vi "Programa_robot_final_6.vi"() -> ()   [LabVIEW 2019]
uses:
  <vilib>/Instr/_visa.llb/VISA Configure Serial Port (Instr).vi
  Global_STOP.vi
  <vilib>/regexp/Match Regular Expression.xnode
panel:
  in  "stop socket 3":bool
  in  "Ruta hacia el fichero que contiene la imagen de la       superficie del ASIC  fotografiada por la camara en el bloque de borrado de la imagen previa capturada":path=path "C:/Trabajo_Robot/Test Asic Javi_2021/Origen Socket SERVO_PCB_BUENO_v5 (muchos asics)/capturaQR.jpg"
  in  "stop 6":bool
  in  "Abrir socket 2":bool
  in  "Cerrar socket 2":bool
  in  "Interruptor Error 2":bool
  in  "stop 5":bool
  out "Datos_QR 3":string
  out "Existe foto anterior?":bool
  in  "STOP TEST 3":bool
  in  "Interruptor Error":bool
  in  "Cerrar socket":bool
  in  "Abrir socket":bool
  out "Error_QR":bool
  out "return count":u32
  out "lectura puerto serie":u32
  out "dato escrito puerto serie":string
  out "TEST OK":bool
  out "error out":errorcluster {"code" format="%f"}
  in  "STOP TEST 2":bool
  out "Datos_QR 2":string
  out "NUMERO ASICS TESTEADOS":i32
  in  "Config File":path=path "C:/Trabajo_Robot/Test Asic Javi_2021/Origen Socket SERVO_PCB_BUENO_v5 (muchos asics)/CONFIG/configuracion_robot_CTAV2022A.test"
  in  "SELECCION DE TEST":string(combo)="COMPLETO"
  in  "?":bool
  out "Boolean":bool
  in  "stop socket 2":bool
  out "Bytes at port 3":u32=1
  in  "IN y":string(combo)="00"
  in  "IN x":string(combo)="00"
  in  "NOK y":string(combo)="00"
  in  "NOK x":string(combo)="00"
  in  "OK y":string(combo)="00"
  in  "OK x":string(combo)="00"
  in  "Operator's name":string(combo)="Juan Rodríguez"
  in  "?":bool
  in  "Fichero de registro":path=path "C:/Trabajo_Robot/Pruebas/Pruebas.txt"
  in  "Path Out Report":path=path "C:/Trabajo_Robot/desde Marzo 2023/Pruebas_PC_APD/RESULT_TEST_C_LABP0/Test_33_ASIC_Referencia"
  in  "stop socket":bool
  out "Bytes at port 1":u32
  out "Iteraciones":i32
  out "Lectura buffer":string="1"
  in  "Delay (ms)":dbl=1.0 min=1.0 max=9.0 step=1.0
  out "Bytes at port 2":u32=1
  in  "Interruptor":bool=TRUE
  in  "stop":bool
  # "SI SE PRESIONA EL BOTON STOP PARA INTERRUMPIR EL TEST,\nHAY QUE APAGAR Y VOLVER A ENCENDER EL ARDUINO\nCON EL SWITCH DE LA CAJA."
  # "x: columna en cada bandeja \ny: fila en cada bandeja"
  # "Funcionamiento: en la primera iteración, el efector se desplaza desde el origen hasta la celda\nintroducida, hace una pausa, va a la posición del socket (0,0), hace otra pausa, va a la celda\nde salida y vuelve al origen. En las iteraciones siguientes hará lo mismo pero recorriendo las\nceldas de la bandeja sucesivamente. Que el desplazamiento se produzca hacia una celda de\nla bandeja OK o de la bandeja NOK depende de la salidad del programa de test de Asics."
types:
  T1 = enum16{"open", "replace", "create", "open or create", "replace or create", "replace or create with confirmation"}
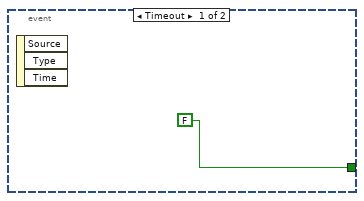
[diagram p2: hidden frame]
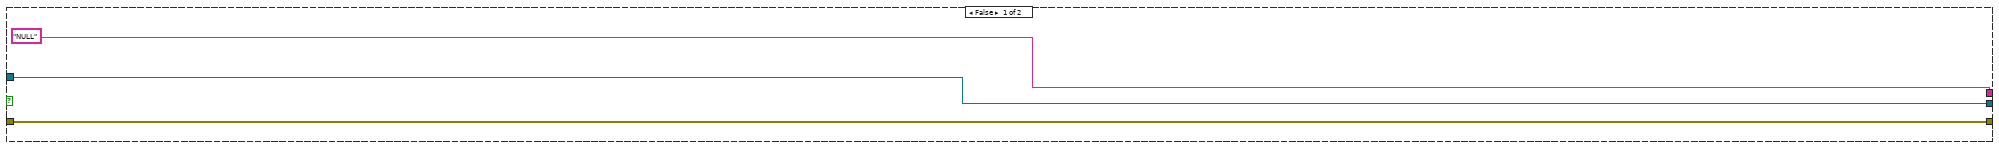
[diagram p5: hidden frame]
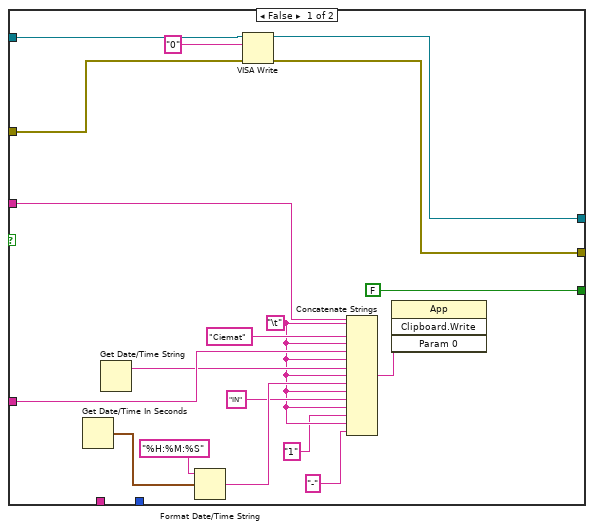
[diagram p9: hidden frame]
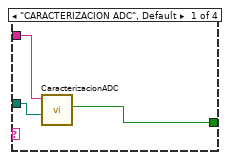
[diagram p10: hidden frame]
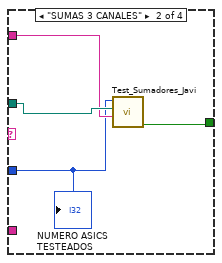
[diagram p11: hidden frame]
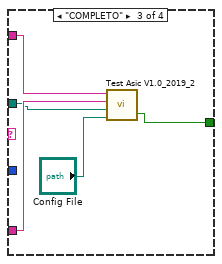
[diagram p12: hidden frame]
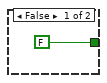
[diagram p13: hidden frame]
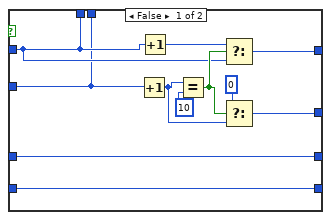
[diagram p15: hidden frame]
diagram:
  n1 = control-ref of="stop socket"() -> (w1:refnum<vi>)
  n2 = control-ref of="Cerrar socket"() -> (w9:refnum<vi>)
  n3 = control-ref of="STOP TEST 2"() -> (w12:refnum<vi>)
  n4 = control-ref of="Abrir socket"() -> (w7:refnum<vi>)
  n5 = control-ref of="stop"() -> (w8:refnum<vi>)
  n6 = control-ref of="Interruptor Error"() -> (w10:refnum<vi>)
  n7 = property class="Bool (strict)"(reference=w12, "Visible"=FALSE) -> ()  [unwired: 1 in, 2 out]
  n8 = property class="Bool (strict)"(reference=w7, "Visible"=FALSE) -> ()  [unwired: 1 in, 2 out]
  n9 = property class="Bool (strict)"(reference=w10, "Visible"=FALSE) -> ()  [unwired: 1 in, 2 out]
  n10 = property class="Bool (strict)"(reference=w9, "Visible"=FALSE) -> ()  [unwired: 1 in, 2 out]
  n11 = property on="Boolean" class="Bool (strict)"("Visible"=FALSE) -> ()  [unwired: 2 in, 2 out]
  n12 = property class="Bool"(reference=w1, "Visible"=FALSE) -> ()  [unwired: 1 in, 2 out]
  n13 = property class="Bool"(reference=w8, "Visible"=FALSE) -> ()  [unwired: 1 in, 2 out]
  n14 = flat-sequence {
    tunnel: [w54] -> w18
    tunnel: ["Fichero de registro"] -> w17
    tunnel: ["SELECCION DE TEST"] -> w16
    tunnel: ["NOK y"] -> w33
    tunnel: ["NOK x"] -> w32
    tunnel: ["OK y"] -> w31
    tunnel: ["OK x"] -> w30
    tunnel: ["IN y"] -> w29
    tunnel: ["IN x"] -> w28
    tunnel: [w57] -> w27
    tunnel: [w58] -> w26
    tunnel: ["IN y"] -> w25
    tunnel: ["IN x"] -> w24
    tunnel: w17 -> [w56]
    frame #0 {
      n15 = while {
        stop <- "?" stop-if-true
        n16 = Not(x="?") -> (.not. x?=w50:bool)
        "Boolean" <- w50
        n17 = property on="Boolean" class="Bool (strict)"("Blinking"=w50) -> ()  [unwired: 2 in, 2 out]
      }
      n18 = global write "Global_STOP.vi" "stop"(FALSE ("stop")) -> ()
    }
    frame #1 {
      n19 = Not(x="?") -> (.not. x?=w54:bool)
    }
    frame #2 {
      n20 = Open/Create/Replace File(file path (use dialog)=w56, operation (0:open)=T1."open", access (0:read/write)=enum16{"read/write", "read-only", "write-only"}."write-only") -> (refnum out=w69:refnum<file>, error out=w71:errorcluster)  [unwired: 3 in, 1 out]
      n21 = Set File Position(refnum=w69, from (0:start)=enum16{"start", "end", "current"}."end", error in=w71) -> (refnum out=w70:refnum<file>, error out=w72:errorcluster)  [unwired: 1 in]
      n22 = Write to Text File(file (use dialog)=w70, text="\r\n", error in=w72) -> (refnum out=w58:refnum<file>, error out=w57:errorcluster)  [unwired: 1 in, 1 out]
    }
  }
  n23 = Decimal String To Number(string=w25) -> (number=w23:i32)  [unwired: 2 in, 1 out]
  n24 = Decimal String To Number(string=w24) -> (number=w20:i32)  [unwired: 2 in, 1 out]
  n25 = Multiply(x=10, y=w23) -> (x*y=w21:i32)
  n26 = Decimal String To Number(string=w31) -> (number=w35:i32)  [unwired: 2 in, 1 out]
  n27 = Decimal String To Number(string=w30) -> (number=w34:i32)  [unwired: 2 in, 1 out]
  n28 = Decimal String To Number(string=w33) -> (number=w37:i32)  [unwired: 2 in, 1 out]
  n29 = Decimal String To Number(string=w32) -> (number=w36:i32)  [unwired: 2 in, 1 out]
  n30 = call-poly "VISA Configure Serial Port"("VISA resource name"=refnum<visa-resource-name> "COM9", "baud rate (9600)"=u32 9600, "data bits (8)"=u16 8) -> ("VISA resource name out"=w41:refnum<visa-resource-name>, "error out"=w44:errorcluster)  [unwired: 11 in]
  n31 = Add(x=w21, y=w20) -> (x+y=w19:i32)
  n32 = while {
    shift-right: [w87] -> w42
    shift-left: w44 -> [w126]
    tunnel: w41 -> [w124]
    tunnel: [w89] -> w43
    tunnel: w26 -> [w117]
    tunnel: [w116] -> w40
    tunnel: w27 -> [w115]
    tunnel: [w114] -> w39
    tunnel: w28 -> [w112]
    tunnel: w29 -> [w111]
    tunnel: w30 -> [w110]
    tunnel: w31 -> [w109]
    tunnel: w32 -> [w108]
    tunnel: w33 -> [w107]
    shift-right: [w100] -> _
    shift-left: w37 -> [w106]
    shift-right: [w102] -> _
    shift-left: w36 -> [w105]
    shift-right: [w99] -> _
    shift-left: w35 -> [w104]
    shift-right: [w101] -> _
    shift-left: w34 -> [w103]
    tunnel: w19 -> [w77]
    tunnel: w18 -> [w91]
    tunnel: w16 -> [w90]
    tunnel: [w78] -> w14
    i -> [w73]
    stop <- w74 stop-if-true
    # "Cuando Arduino deja un ASIC en la bandeja de  entrada ó en las de OK/NOK\ny vuelve a la posicion de socket, envia un \"2\" por el puerto serie\na labview y éste lo lee para que se salga del bucle, y prosiga la secuencia que le queda\nal programa, para después coger otro asic. Javier Morales"
    n33 = flat-sequence {
      tunnel: w126 -> [w179]
      tunnel: w124 -> [w168]
      tunnel: [w170] -> w123
      tunnel: [w169] -> w122
      tunnel: w112 -> [w149]
      tunnel: w111 -> [w148]
      tunnel: w110 -> [w147]
      tunnel: w109 -> [w146]
      tunnel: w108 -> [w145]
      tunnel: w107 -> [w144]
      tunnel: w123 -> [w916]
      tunnel: w122 -> [w915]
      tunnel: [w914] -> w98
      tunnel: [w913] -> w96
      tunnel: [w912] -> _
      tunnel: w98 -> [w933]
      tunnel: [w931] -> w97
      tunnel: w96 -> [w932]
      tunnel: [w930] -> w95
      tunnel: w97 -> [w954]
      tunnel: w95 -> [w953]
      tunnel: w73 -> [w955]
      tunnel: [w951] -> w94
      tunnel: [w950] -> w93
      tunnel: [w949] -> w92
      tunnel: w73 -> [w1071]
      tunnel: [w1073] -> w120
      tunnel: [w1072] -> w119
      tunnel: [w1069] -> w113
      tunnel: w94 -> [w1068]
      tunnel: w93 -> [w1067]
      tunnel: w92 -> [w1066]
      tunnel: w91 -> [w1061]
      tunnel: w90 -> [w1064]
      tunnel: w73 -> [w1063]
      tunnel: [w1141] -> w118
      tunnel: [w1143] -> w121
      tunnel: w120 -> [w1142]
      tunnel: w119 -> [w1140]
      tunnel: w117 -> [w1147]
      tunnel: [w1146] -> w116
      tunnel: w115 -> [w1145]
      tunnel: [w1144] -> w114
      tunnel: w73 -> [w1137]
      tunnel: w113 -> [w1136]
      tunnel: w106 -> [w1132]
      tunnel: w105 -> [w1135]
      tunnel: w104 -> [w1134]
      tunnel: w103 -> [w1133]
      tunnel: [w1131] -> w100
      tunnel: [w1130] -> w102
      tunnel: [w1129] -> w99
      tunnel: [w1128] -> w101
      tunnel: w77 -> [w1127]
      tunnel: w73 -> [w1126]
      tunnel: [w1125] -> _
      frame #0 {
        n34 = for {
          N: 2 -> [_]
          shift-right: [w791] -> _
          shift-left: w149 -> [w796]
          shift-right: [w794] -> w165
          shift-left: w168 -> [w795]
          shift-right: [w792] -> w164
          shift-left: w179 -> [w793]
          n35 = xnode "Match Regular Expression"("input string"=w796, "regular expression"="-?\\d") -> ("whole match"=w790:string, "after match"=w791:string)  [unwired: 4 in, 3 out]
          n36 = VISA Write(VISA resource name=w795, write buffer=w790, error in (no error)=w793) -> (VISA resource name out=w794:refnum<visa-resource-name>, error out=w792:errorcluster)  [unwired: 1 out]
        }
        n37 = for {
          N: 2 -> [_]
          shift-right: [w669] -> _
          shift-left: w148 -> [w674]
          shift-right: [w672] -> w159
          shift-left: w165 -> [w673]
          shift-right: [w670] -> w158
          shift-left: w164 -> [w671]
          n38 = xnode "Match Regular Expression"("input string"=w674, "regular expression"="-?\\d") -> ("whole match"=w668:string, "after match"=w669:string)  [unwired: 4 in, 3 out]
          n39 = VISA Write(VISA resource name=w673, write buffer=w668, error in (no error)=w671) -> (VISA resource name out=w672:refnum<visa-resource-name>, error out=w670:errorcluster)  [unwired: 1 out]
        }
        n40 = for {
          N: 2 -> [_]
          shift-right: [w547] -> _
          shift-left: w147 -> [w552]
          shift-right: [w550] -> w161
          shift-left: w159 -> [w551]
          shift-right: [w548] -> w160
          shift-left: w158 -> [w549]
          n41 = xnode "Match Regular Expression"("input string"=w552, "regular expression"="-?\\d") -> ("whole match"=w546:string, "after match"=w547:string)  [unwired: 4 in, 3 out]
          n42 = VISA Write(VISA resource name=w551, write buffer=w546, error in (no error)=w549) -> (VISA resource name out=w550:refnum<visa-resource-name>, error out=w548:errorcluster)  [unwired: 1 out]
        }
        n43 = for {
          N: 2 -> [_]
          shift-right: [w425] -> _
          shift-left: w146 -> [w430]
          shift-right: [w428] -> w153
          shift-left: w161 -> [w429]
          shift-right: [w426] -> w152
          shift-left: w160 -> [w427]
          n44 = xnode "Match Regular Expression"("input string"=w430, "regular expression"="-?\\d") -> ("whole match"=w424:string, "after match"=w425:string)  [unwired: 4 in, 3 out]
          n45 = VISA Write(VISA resource name=w429, write buffer=w424, error in (no error)=w427) -> (VISA resource name out=w428:refnum<visa-resource-name>, error out=w426:errorcluster)  [unwired: 1 out]
        }
        n46 = for {
          N: 2 -> [_]
          shift-right: [w303] -> _
          shift-left: w145 -> [w308]
          shift-right: [w306] -> w155
          shift-left: w153 -> [w307]
          shift-right: [w304] -> w154
          shift-left: w152 -> [w305]
          n47 = xnode "Match Regular Expression"("input string"=w308, "regular expression"="-?\\d") -> ("whole match"=w302:string, "after match"=w303:string)  [unwired: 4 in, 3 out]
          n48 = VISA Write(VISA resource name=w307, write buffer=w302, error in (no error)=w305) -> (VISA resource name out=w306:refnum<visa-resource-name>, error out=w304:errorcluster)  [unwired: 1 out]
        }
        n49 = for {
          N: 2 -> [_]
          shift-right: [w181] -> _
          shift-left: w144 -> [w186]
          shift-right: [w184] -> w151
          shift-left: w155 -> [w185]
          shift-right: [w182] -> w150
          shift-left: w154 -> [w183]
          n50 = xnode "Match Regular Expression"("input string"=w186, "regular expression"="-?\\d") -> ("whole match"=w180:string, "after match"=w181:string)  [unwired: 4 in, 3 out]
          n51 = VISA Write(VISA resource name=w185, write buffer=w180, error in (no error)=w183) -> (VISA resource name out=w184:refnum<visa-resource-name>, error out=w182:errorcluster)  [unwired: 1 out]
        }
        n52 = Number To Decimal String(number="Delay (ms)") -> (decimal integer string=w173:string)  [unwired: 1 in]
        n53 = VISA Write(VISA resource name=w151, write buffer=w173, error in (no error)=w150) -> (VISA resource name out=w175:refnum<visa-resource-name>, error out=w174:errorcluster)  [unwired: 1 out]
        n54 = Select(t="1" ("write buffer"), s="Interruptor", f="0" ("write buffer")) -> (s? t:f=w171:string)
        n55 = VISA Write(VISA resource name=w175, write buffer=w171, error in (no error)=w174) -> (VISA resource name out=w170:refnum<visa-resource-name>, error out=w169:errorcluster)  [unwired: 1 out]
      }
      frame #1 {
        n56 = while {
          shift-right: [w923] -> w913
          shift-left: w915 -> [w928]
          tunnel: ["stop socket"] -> _
          shift-right: [w924] -> w914
          shift-left: w916 -> [w929]
          tunnel: ["stop socket"] -> w912
          stop <- w918 stop-if-true
          n57 = property class="Instr"(reference=w929, error in=w928) -> (reference out=w927:refnum<visa-resource-name>, error out=w926:errorcluster, "Bytes at Port"=w925:u32)
          "Bytes at port 1" <- w925
          n58 = VISA Read(VISA resource name=w927, byte count=w925, error in (no error)=w926) -> (VISA resource name out=w924:refnum<visa-resource-name>, read buffer=w922:string, error out=w923:errorcluster)  [unwired: 1 out]
          n59 = Equal?(x="2", y=w922) -> (x = y?=w920:bool)
          n60 = global read "Global_STOP.vi" "stop"() -> (w917:bool)
          n61 = Compound Arithmetic op=OR(w920, "stop socket", w917) -> (w918:bool)
        }
      }
      frame #2 {
        n62 = while {
          shift-right: [w940] -> w930
          shift-left: w932 -> [w945]
          tunnel: ["stop socket 2"] -> _
          shift-right: [w941] -> w931
          shift-left: w933 -> [w946]
          tunnel: ["stop socket 2"] -> _
          stop <- w935 stop-if-true
          n63 = property class="Instr"(reference=w946, error in=w945) -> (reference out=w944:refnum<visa-resource-name>, error out=w943:errorcluster, "Bytes at Port"=w942:u32)
          "Bytes at port 3" <- w942
          n64 = VISA Read(VISA resource name=w944, byte count=w942, error in (no error)=w943) -> (VISA resource name out=w941:refnum<visa-resource-name>, read buffer=w939:string, error out=w940:errorcluster)  [unwired: 1 out]
          n65 = Equal?(x="3", y=w939) -> (x = y?=w937:bool)
          n66 = global read "Global_STOP.vi" "stop"() -> (w934:bool)
          n67 = Compound Arithmetic op=OR(w937, "stop socket 2", w934) -> (w935:bool)
        }
      }
      frame #3 {
        # "Este bloque realiza la captura y lectura del QR"
        n68 = Greater?(x=w955, y=-1) -> (0:w952:bool)
        n69 = case shown="True" w952 {
          tunnel: [w959 w962] -> w949
          tunnel: w954 -> [w959 w964]
          tunnel: [w958 w963] -> w951
          tunnel: w953 -> [w958 w965]
          tunnel: ["NULL" ("Datos_QR") w961] -> w950
          frame False {
          }
          frame True {
            n70 = property on="Error_QR" class="Bool (strict)"("Value"=FALSE ("Error_QR")) -> ()  [unwired: 2 in, 2 out]
            n71 = while {
              tunnel: [w972] -> w961
              tunnel: w964 -> [w982]
              tunnel: [w978] -> w962
              tunnel: [w977] -> w963
              tunnel: w965 -> [w973]
              stop <- w970 stop-if-true
              n72 = flat-sequence {
                tunnel: [w986] -> w974
                tunnel: w973 -> [w984]
                tunnel: [w998] -> w972
                tunnel: [w997] -> w967
                tunnel: w974 -> [w996]
                tunnel: [w996] -> w968
                frame #0 {
                  # "Éste bloque borra el fichero de imagen\ndel Asic anterior."
                  n73 = call <vilib>:"Check if File or Folder Exists.vi"("error in (no error)"=w984, "path"="Ruta hacia el fichero que contiene la imagen de la       superficie del ASIC  fotografiada por la camara en el bloque de borrado de la imagen previa capturada") -> ("error out"=w985:errorcluster, "file or folder exists?"=w988:bool, "dup path"=w987:path)  [unwired: 7 in]
                  "Existe foto anterior?" <- w988
                  n74 = case shown="True" w988 {
                    tunnel: w987 -> [w990 w994]
                    tunnel: [w990 w993] -> _
                    tunnel: [w989 w992] -> w986
                    tunnel: w985 -> [w989 w991]
                    frame False {
                    }
                    frame True {
                      n75 = Delete(path (use dialog)=w994, error in=w991) -> (deleted path=w993:path, error out=w992:errorcluster)  [unwired: 3 in, 1 out]
                    }
                  }
                }
                frame #1 {
                  # "Éste bloque realiza la captura de imagen\ndel QR del Asic para leer el código."
                  n76 = for {
                    N: 5 -> [_]
                    tunnel: [w1003] -> w998
                    tunnel: [w1001] -> w997
                    stop <- w999 stop-if-true
                    n77 = call "CapturaImagenyQR_subVI_pruebas.vi"() -> ("Datos_QR"=w1003:string)  [unwired: 11 in]
                    "Datos_QR 3" <- w1003
                    n78 = Equal?(x=w1003, y="" ("Datos_QR")) -> (x = y?=w1002:bool)
                    n79 = global read "Global_STOP.vi" "stop"() -> (w1000:bool)
                    n80 = Not(x=w1002) -> (.not. x?=w1001:bool)
                    n81 = Compound Arithmetic op=OR(w1001, w1000) -> (w999:bool)
                  }
                }
              }
              n82 = Not(x=w967) -> (.not. x?=w969:bool)
              "Error_QR" <- w969
              n83 = Select(t="1" ("write buffer"), s=w967, f="0" ("write buffer")) -> (s? t:f=w979:string)
              n84 = VISA Write(VISA resource name=w982, write buffer=w979, error in (no error)=w968) -> (VISA resource name out=w976:refnum<visa-resource-name>, error out=w975:errorcluster)  [unwired: 1 out]
              n85 = global read "Global_STOP.vi" "stop"() -> (w971:bool)
              n86 = case shown="False" w967 {
                tunnel: w976 -> [w1016 w1057]
                tunnel: w975 -> [w1015 w1056]
                tunnel: [w1014 w1057] -> w978
                tunnel: [w1013 w1056] -> w977
                frame False {
                  n87 = flat-sequence {
                    tunnel: w1016 -> [w1020]
                    tunnel: [w1019] -> w1012
                    tunnel: [w1018] -> w1010
                    tunnel: w1015 -> [w1017]
                    tunnel: w1012 -> [w1033]
                    tunnel: [w1033] -> w1011
                    tunnel: w1010 -> [w1032]
                    tunnel: [w1032] -> w1009
                    tunnel: w1011 -> [w1037]
                    tunnel: w1009 -> [w1036]
                    tunnel: [w1035] -> w1008
                    tunnel: [w1034] -> w1006
                    tunnel: w1008 -> [w1050]
                    tunnel: [w1050] -> w1007
                    tunnel: w1006 -> [w1049]
                    tunnel: [w1049] -> w1005
                    tunnel: [w1051] -> w1013
                    tunnel: [w1052] -> w1014
                    tunnel: w1007 -> [w1052]
                    tunnel: w1005 -> [w1051]
                    frame #0 {
                      n88 = while {
                        tunnel: w1020 -> [w1030]
                        tunnel: [w1026] -> w1019
                        tunnel: [w1025] -> w1018
                        tunnel: w1017 -> [w1024]
                        stop <- w1021 stop-if-true
                        n89 = global read "Global_STOP.vi" "stop"() -> (w1023:bool)
                        n90 = Select(t="2" ("write buffer"), s="Abrir socket", f="0" ("write buffer")) -> (s? t:f=w1027:string)
                        n91 = Or(x=w1023, y="Abrir socket") -> (x .or. y?=w1021:bool)
                        n92 = VISA Write(VISA resource name=w1030, write buffer=w1027, error in (no error)=w1024) -> (VISA resource name out=w1026:refnum<visa-resource-name>, error out=w1025:errorcluster)  [unwired: 1 out]
                      }
                    }
                    frame #1 {
                      n93 = Wait (ms)(milliseconds to wait=u32 1000) -> ()  [unwired: 1 out]
                    }
                    frame #2 {
                      n94 = while {
                        tunnel: w1037 -> [w1044]
                        tunnel: w1036 -> [w1043]
                        tunnel: [w1042] -> w1035
                        tunnel: [w1041] -> w1034
                        stop <- w1040 stop-if-true
                        n95 = global read "Global_STOP.vi" "stop"() -> (w1039:bool)
                        n96 = Select(t="3" ("write buffer"), s="Cerrar socket", f="0" ("write buffer")) -> (s? t:f=w1045:string)
                        n97 = Or(x=w1039, y="Cerrar socket") -> (x .or. y?=w1040:bool)
                        n98 = VISA Write(VISA resource name=w1044, write buffer=w1045, error in (no error)=w1043) -> (VISA resource name out=w1042:refnum<visa-resource-name>, error out=w1041:errorcluster)  [unwired: 1 out]
                      }
                    }
                    frame #3 {
                      n99 = Wait (ms)(milliseconds to wait=u32 1000) -> ()  [unwired: 1 out]
                    }
                    frame #4 {
                      n100 = while {
                        stop <- w1053 stop-if-true
                        n101 = global read "Global_STOP.vi" "stop"() -> (w1055:bool)
                        n102 = Or(x="Interruptor Error", y=w1055) -> (x .or. y?=w1053:bool)
                      }
                    }
                  }
                }
                frame True {
                }
              }
              n103 = Or(x=w967, y=w971) -> (x .or. y?=w970:bool)
              n104 = case shown="True" w969 {
                frame False {
                }
                frame True {
                  n105 = call "Send Email"() -> ()  [unwired: 11 in, 1 out]
                }
              }
            }
            n106 = Wait (ms)(milliseconds to wait=u32 10000) -> ()  [unwired: 1 out]
          }
        }
        n107 = control-ref of="STOP TEST 2"() -> (w948:refnum<vi>)
        n108 = property class="Bool (strict)"(reference=w948, "Visible"=TRUE) -> ()  [unwired: 1 in, 2 out]
      }
      frame #4 {
        n109 = global read "Global_STOP.vi" "stop"() -> (w1060:bool)
        n110 = Greater?(x=w1071, y=-1) -> (0:w1062:bool)
        n111 = Not(x=w1060) -> (.not. x?=w1059:bool)
        n112 = Compound Arithmetic op=AND(w1062, w1061, w1059) -> (w1058:bool)
        n113 = case shown="True" w1058 {
          tunnel: w1066 -> [w1089 w1097]
          tunnel: w1068 -> [w1088 w1096]
          tunnel: [w1087 w1095] -> w1073
          tunnel: [w1086 w1094] -> w1072
          tunnel: w1067 -> [w1082 w1103]
          tunnel: [FALSE ("Boolean") w1101] -> w1069
          tunnel: "Operator's name" -> [w1080 w1100]
          tunnel: w1064 -> [_ w1092]
          tunnel: w1063 -> [_ w1099]
          frame False {
            w1076 = "\t"
            n114 = Get Date/Time In Seconds() -> (seconds since 1Jan1904=w1084:timestamp)
            n115 = Get Date/Time String() -> (date string=w1079:string)  [unwired: 3 in, 1 out]
            n116 = Format Date/Time String(time format string (%c)="%H:%M:%S", seconds (now)=w1084) -> (date/time string=w1078:string)  [unwired: 1 in]
            n117 = VISA Write(VISA resource name=w1089, write buffer="0", error in (no error)=w1088) -> (VISA resource name out=w1087:refnum<visa-resource-name>, error out=w1086:errorcluster)  [unwired: 1 out]
            n118 = Concatenate Strings(w1082, w1076, "Ciemat", w1076, w1080, w1076, w1079, w1076, w1078, w1076, "IN", w1076, "1", w1076, "-") -> (w1085:string)
            n119 = invoke class="App" method="Clipboard.Write"("Param 0"=w1085) -> ()  [unwired: 3 in, 4 out]
          }
          frame True {
            # "Test de Asics"
            n120 = case shown="\"SOLO MOVIMIENTO\"" w1092 {
              tunnel: w1103 -> [w1108 w1110 w1117 _]
              tunnel: "Path Out Report" -> [w1107 w1112 w1115 _]
              tunnel: [w1106 w1111 w1113 w1118] -> w1101
              tunnel: w1100 -> [_ _ w1116 _]
              tunnel: w1099 -> [_ w1109 _ w1122]
              frame "CARACTERIZACION ADC", Default {
                n121 = call "CaracterizacionADC.vi"("QR code"=w1108, "Path Out Report"=w1107) -> ("OK/NOK"=w1106:bool)  [unwired: 7 in]
              }
              frame "SUMAS 3 CANALES" {
                n122 = call "Test_Sumadores_Javi.vi"("QR"=w1110, "Path"=w1112, "NUMERO DE PASADA DE TEST"=w1109) -> ("Boolean"=w1111:bool)  [unwired: 8 in]
                "NUMERO ASICS TESTEADOS" <- w1109
              }
              frame "COMPLETO" {
                n123 = call "Test Asic V1.0_2019_2.vi"("Config File"="Config File", "Path Out Report"=w1115, "Operator's Name"=w1116, "ASIC'S Number"=w1117) -> ("OK, Fault 2"=w1113:bool)  [unwired: 1 in]
              }
              frame "SOLO MOVIMIENTO" {
                n124 = Quotient & Remainder(x=w1122, y=2) -> (x-y*floor(x/y)=w1119:i32)  [unwired: 1 out]
                n125 = Equal To 0?(x=w1119) -> (x = 0?=w1120:bool)
                n126 = case shown="True" w1120 {
                  tunnel: [FALSE FALSE] -> w1118
                  frame False {
                  }
                  frame True {
                  }
                }
              }
            }
            "TEST OK" <- w1101
            n127 = Select(t="1" ("write buffer"), s=w1101, f="0" ("write buffer")) -> (s? t:f=w1098:string)
            "dato escrito puerto serie" <- w1098
            n128 = VISA Write(VISA resource name=w1097, write buffer=w1098, error in (no error)=w1096) -> (VISA resource name out=w1095:refnum<visa-resource-name>, return count=→"return count":u32, error out=w1094:errorcluster)
          }
        }
      }
      frame #5 {
        n129 = Greater?(x=w1137, y=-1) -> (0:w1138:bool)
        n130 = case shown="True" w1138 {
          tunnel: w1147 -> [w1153 w1186]
          tunnel: [w1153 w1185] -> w1146
          tunnel: w1145 -> [w1152 w1184]
          tunnel: [w1152 w1183] -> w1144
          tunnel: [w1155 w1182] -> w1143
          tunnel: w1142 -> [w1155 w1182]
          tunnel: [w1154 w1181] -> w1141
          tunnel: w1140 -> [w1154 w1181]
          tunnel: w1136 -> [_ w1179]
          tunnel: w1132 -> [w1151 w1178]
          tunnel: w1135 -> [w1150 w1177]
          tunnel: w1134 -> [w1149 w1176]
          tunnel: w1133 -> [w1148 w1175]
          tunnel: [w1151 w1174] -> w1131
          tunnel: [w1150 w1173] -> w1130
          tunnel: [w1149 w1172] -> w1129
          tunnel: [w1148 w1171] -> w1128
          frame False {
          }
          frame True {
            w1158 = "\t"
            # "Registro de datos en fichero"
            n131 = invoke class="App" method="Clipboard.Read"() -> ("Read Clipbrd"=w1180:string)  [unwired: 3 in, 2 out]
            n132 = case shown="True" w1179 {
              tunnel: w1178 -> [w1189 w1202]
              tunnel: w1177 -> [w1188 w1201]
              tunnel: w1176 -> [w1191 w1199]
              tunnel: w1175 -> [w1190 w1200]
              tunnel: [w1193 w1202] -> w1174
              tunnel: [w1192 w1201] -> w1173
              tunnel: [w1191 w1204] -> w1172
              tunnel: [w1190 w1203] -> w1171
              tunnel: [w1189 w1199] -> w1170
              tunnel: [w1188 w1200] -> w1169
              frame False {
                n133 = Increment(x=w1188) -> (x+1=w1197:i32)
                n134 = Increment(x=w1189) -> (x+1=w1194:i32)
                n135 = Equal?(x=w1197, y=10) -> (x = y?=w1195:bool)
                n136 = Select(t=w1194, s=w1195, f=w1189) -> (s? t:f=w1193:i32)
                n137 = Select(t=0, s=w1195, f=w1197) -> (s? t:f=w1192:i32)
              }
              frame True {
                n138 = Increment(x=w1200) -> (x+1=w1208:i32)
                n139 = Increment(x=w1199) -> (x+1=w1205:i32)
                n140 = Equal?(x=w1208, y=10) -> (x = y?=w1206:bool)
                n141 = Select(t=w1205, s=w1206, f=w1199) -> (s? t:f=w1204:i32)
                n142 = Select(t=0, s=w1206, f=w1208) -> (s? t:f=w1203:i32)
              }
            }
            n143 = Write to Text File(file (use dialog)=w1186, text=w1180, error in=w1184) -> (refnum out=w1167:refnum<file>, error out=w1168:errorcluster)  [unwired: 1 in, 1 out]
            n144 = Number To Decimal String(number=w1170) -> (decimal integer string=w1157:string)  [unwired: 1 in]
            n145 = Number To Decimal String(number=w1169) -> (decimal integer string=w1156:string)  [unwired: 1 in]
            n146 = Write to Text File(file (use dialog)=w1167, text=w1158, error in=w1168) -> (refnum out=w1165:refnum<file>, error out=w1166:errorcluster)  [unwired: 1 in, 1 out]
            n147 = Write to Text File(file (use dialog)=w1165, text=w1157, error in=w1166) -> (refnum out=w1162:refnum<file>, error out=w1161:errorcluster)  [unwired: 1 in, 1 out]
            n148 = Write to Text File(file (use dialog)=w1162, text=w1158, error in=w1161) -> (refnum out=w1160:refnum<file>, error out=w1159:errorcluster)  [unwired: 1 in, 1 out]
            n149 = Write to Text File(file (use dialog)=w1160, text=w1156, error in=w1159) -> (refnum out=w1164:refnum<file>, error out=w1163:errorcluster)  [unwired: 1 in, 1 out]
            n150 = Write to Text File(file (use dialog)=w1164, text="\r\n", error in=w1163) -> (refnum out=w1185:refnum<file>, error out=w1183:errorcluster)  [unwired: 1 in, 1 out]
          }
        }
        n151 = Add(x=w1127, y=w1126) -> (x+y=w1125:i32)
      }
    }
    n152 = while {
      shift-right: [w1217] -> w82
      shift-left: w118 -> [w1223]
      tunnel: ["stop"] -> _
      shift-right: [w1218] -> w89
      shift-left: w121 -> [w1224]
      tunnel: [w1213] -> w125
      stop <- w1211 stop-if-true
      # "1"
      n153 = property class="Instr"(reference=w1224, error in=w1223) -> (reference out=w1221:refnum<visa-resource-name>, error out=w1220:errorcluster, "Bytes at Port"=w1219:u32)
      "Bytes at port 2" <- w1219
      n154 = VISA Read(VISA resource name=w1221, byte count=w1219, error in (no error)=w1220) -> (VISA resource name out=w1218:refnum<visa-resource-name>, read buffer=w1213:string, return count=w1216:u32, error out=w1217:errorcluster)
      "lectura puerto serie" <- w1216
      n155 = Greater Or Equal?(x=w1216, y=u32 1) -> (x >= y?=w1214:bool)
      n156 = global read "Global_STOP.vi" "stop"() -> (w1210:bool)
      n157 = Or(x=w1214, y="stop") -> (x .or. y?=w1212:bool)
      n158 = Compound Arithmetic op=OR(w1212, w1210) -> (w1211:bool)
    }
    "Lectura buffer" <- w125
    n159 = flat-sequence {
      tunnel: w82 -> [w128]
      tunnel: [w128] -> w81
      tunnel: [w127] -> w79
      frame #0 {
        n160 = global read "Global_STOP.vi" "stop"() -> (w127:bool)
      }
    }
    n161 = Greater?(x=w73, y=163) -> (0:w75:bool)
    n162 = case shown="False" w79 {
      selector: w79 -> [_ w138]
      tunnel: [w132 _] -> w86
      tunnel: [w129 w138] -> w83
      tunnel: w81 -> [w130 w137]
      tunnel: [w130 w137] -> w80
      frame False {
        n163 = for {
          N: 3 -> [_]
          tunnel: [w135] -> _
          tunnel: [w133] -> w132
          tunnel: [w133] -> w129
          stop <- w133 stop-if-true
          n164 = call "CapturaImagenyQR_subVI.vi"() -> ("Datos_QR"=w135:string)  [unwired: 11 in]
          "Datos_QR 2" <- w135
          n165 = Equal?(x=w135, y="" ("Datos_QR")) -> (x = y?=w134:bool)
          n166 = Not(x=w134) -> (.not. x?=w133:bool)
        }
      }
      frame True {
      }
    }
    n167 = flat-sequence {
      tunnel: [w141] -> w78
      tunnel: w83 -> [w139]
      frame #0 {
        n168 = global read "Global_STOP.vi" "stop"() -> (w140:bool)
        n169 = Or(x=w139, y=w140) -> (x .or. y?=w141:bool)
      }
    }
    n170 = Boolean To (0,1)(Boolean=w86) -> (0, 1=w85:i16)
    n171 = call <vilib>:"Error Cluster From Error Code.vi"("error in (no error)"=w80, "error message (\"\")"="El asic no se ha colocado en la\n    bandeja de salida,se ha quedado\nen el socket posiblemente por una\nmala succión de la ventosa.\nPresione STOP\n" ("error message (\"\")"), "error code (0)"=w85) -> ("error out"=w84:errorcluster)  [unwired: 6 in]
    n172 = call <vilib>:"Simple Error Handler.vi"("error in (no error)"=w84) -> ("error out"=w87:errorcluster)  [unwired: 4 in, 4 out]
    n173 = Or(x=w78, y=w75) -> (x .or. y?=w74:bool)
    n174 = case shown="True" w86 {
      selector: w86 -> [w142 w143]
      tunnel: [w142 w143] -> _
      frame False {
      }
      frame True {
        n175 = call "Send Email2"() -> ()  [unwired: 11 in, 1 out]
      }
    }
    "Iteraciones" <- w73
  }
  n176 = flat-sequence {
    frame #0 {
      n177 = local write "STOP TEST 2"(FALSE ("STOP TEST 2")) -> ()
    }
    frame #1 {
      n178 = while {
        stop <- w1226 stop-if-true
        n179 = event shown="[1] \"STOP TEST 2\": Value Change" {
          selector: _ -> [_ _]
          dyn-events: _ -> [_ _]
          timeout: _ -> [_ _]
          tunnel: [FALSE "STOP TEST 2"] -> w1226
          event Timeout {
            n180 = event-data() -> ()  [unwired: 1 in, 3 out]
          }
          event "STOP TEST 2": Value Change {
            n181 = event-data() -> ()  [unwired: 1 in, 6 out]
            n182 = global write "Global_STOP.vi" "stop"("STOP TEST 2") -> ()
            n183 = Wait (ms)(milliseconds to wait=u32 100) -> ()  [unwired: 1 out]
          }
        }
      }
    }
  }
  n184 = Close File(refnum=w40, error in=w39) -> (error out=w38:errorcluster)  [unwired: 1 out]
  n185 = Not(x=w14) -> (.not. x?=w15:bool)
  n186 = call <vilib>:"Simple Error Handler.vi"("error in (no error)"=w38) -> ()  [unwired: 4 in, 5 out]
  n187 = global write "Global_STOP.vi" "stop"(w15) -> ()
  n188 = VISA Close(VISA resource name=w43, error in (no error)=w42) -> (error out=→"error out":errorcluster)
